vi "PH_ImageCalibrator.set User Dialog.vi"(0 "i ref in":refnum<vi>, 2 "State":string, 3 "Text":string, 5 "error in (no error)":errorcluster) -> (14 "i ref out":refnum<vi>, 19 "error out":errorcluster)   [LabVIEW 2014, in "PH_ImageCalibrator.lvlib"]
doc: "This VI sets the User Dialog"
uses:
  PH_ImageCalibrator.lvlib
  PH_Common/PH_Common.lvlib
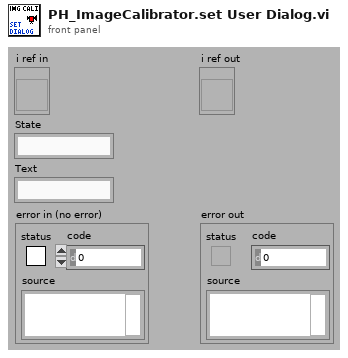
[diagram p1: front panel]
types:
  T1 = typedef "PH_ImageCalibrator.lvlib/PH_ImageCalibrator.i attribute.ctl" = cluster{"GUI Refs":cluster{"Available Cams":refnum<vi>, "OK":refnum<vi>, "Skip":refnum<vi>, "Repeat":refnum<vi>, "Cancel":refnum<vi>, "Length [mm]":refnum<vi>, "Energy [mJ]":refnum<vi>, "Dialog":refnum<vi>}, "Cam instances":string[], "Dark Pics":cluster{"#":i32, "BI taken":bool}, "Lin Cali":cluster{"Distance [Pixel]":dbl, "Distance [mm]":dbl, "Lin Cali Factor [mm/Pixel]":dbl}, "Energy Cali":cluster{"Pixelsum":dbl, "Energy [mJ]":dbl, "Energy Cali factor [mJ/Pixelsum]":dbl, "Underground subtracted?":bool, "#":i32}, "Images":cluster{"Background":T2, "Energy":T2}}
  T2 = typedef "IMAQ Image.ctl" = refnum<image>
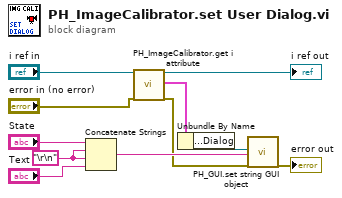
[diagram p0: block diagram]
diagram:
  w1 = "\r\n"
  n1 = Concatenate Strings("State", w1, w1, "Text") -> (w5:string)
  n2 = call "PH_ImageCalibrator.get i attribute.vi"("i ref in"="i ref in", "error in (no error)"="error in (no error)") -> ("i ref out"=→"i ref out":refnum<vi>, "i attribute"=w6:T1, "error out"=w3:errorcluster)  [unwired: 15 in]
  n3 = Unbundle By Name(w6) -> ("GUI Refs.Dialog"=w4:refnum<vi>)
  n4 = call "PH_GUI.set string GUI object.vi"("GUI object Ref"=w4, "Text"=w5, "error in"=w3) -> ("error out"=→"error out":errorcluster)  [unwired: 16 in]
